vi "Juicer-CloseAll.vi"(7 "Device reference":refnum<vi>, 8 "error in (no error)":errorcluster, 9 "Eventstring":string="auto-generate") -> (0 "error out":errorcluster)   [LabVIEW 2011]
doc: "Closes all juicer valves.\n\nDevice reference: which juicer?\nEventstring: used for timestamping\n--empty: no timestamp will be generated\n--unwired or \"auto-generate\": TS w/ default eventstring\n--otherwise: TS with user-provided string\n\nThe default eventstring is:\n[juicer name].closeAll\nwhere [juicer name] is the referenced juicer's front panel label text.\n\nThis just calls Juicer-Close for each valve in sequence (from 1-12). A timestamp is only generated at the last valve."
uses:
  Typedefs/Juicer.ctl
  Rack/Typedefs/OutputRequest.ctl
  Rack/Typedefs/OutputRequest refnum.ctl
  Rack/Methods/Port drivers/DigitalInput-DataCluster.ctl
  Rack/Typedefs/InputData cluster.ctl
panel:
  # "(must be on same NI card)"
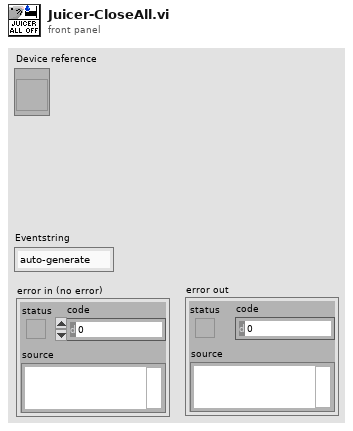
[diagram p1: front panel]
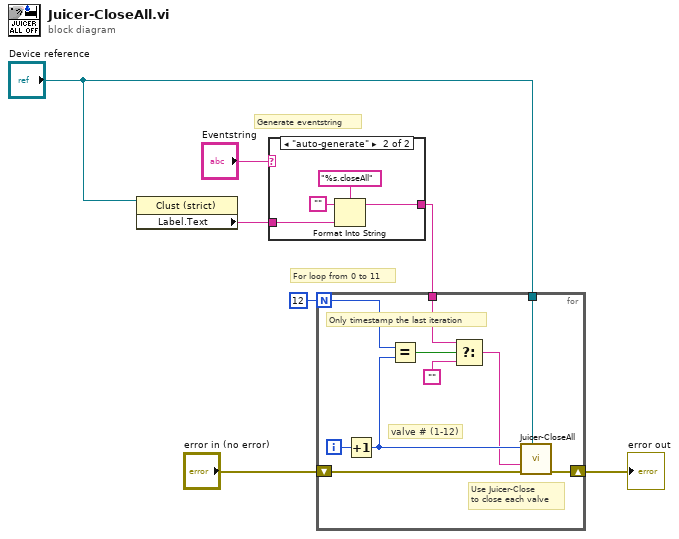
[diagram p0: block diagram]
diagram:
  # "Generate eventstring"
  # "For loop from 0 to 11"
  n1 = property class="Clust (strict)"(reference="Device reference") -> ("Label.Text"=w5:string)  [unwired: 1 in, 2 out]
  n2 = case shown="\"auto-generate\"" "Eventstring" {
    selector: "Eventstring" -> [w8 _]
    tunnel: [w8 w10] -> w4
    tunnel: w5 -> [_ w9]
    frame Default {
      # "Use user-provided string"
    }
    frame "auto-generate" {
      n3 = Format Into String(format string="%s.closeAll", initial string="", w9) -> (resulting string=w10:string)  [unwired: 1 in, 1 out]
    }
  }
  n4 = for {
    N: 12 -> [w21]
    tunnel: w4 -> [w19]
    tunnel: "Device reference" -> [w14]
    shift-right: [w13] -> w1
    shift-left: "error in (no error)" -> [w16]
    i -> [w22]
    # "Use Juicer-Close\nto close each valve"
    # "valve # (1-12)"
    # "Only timestamp the last iteration"
    n5 = Increment(x=w22) -> (x+1=w17:i32)
    n6 = Equal?(x=w21, y=w17) -> (x = y?=w20:bool)
    n7 = Select(t=w19, s=w20, f="") -> (s? t:f=w15:string)
    n8 = call "Juicer-CloseAll.vi"("Device reference"=w14, "error in (no error)"=w16, "Eventstring"=w15, 11:w17) -> ("error out"=w13:errorcluster)  [unwired: 7 in]
  }
  "error out" <- w1
